vi "SMO.StopDependencies.vi"(8 "error in (no error)":errorcluster, 11 "SMO in":refnum<class "SMO.lvclass">) -> (0 "error out":errorcluster, 3 "SMO out":refnum<class "SMO.lvclass">)   [LabVIEW 2021, in "smo.lvlib" / "SMO.lvclass"]
uses:
  SMO.lvclass
  SMO.lvclass/SMO.ctl
  Typedefs/SMO Dependency Event--Cluster.ctl
  Typedefs/SMO Dependency Event--Enum.ctl
  GetVariant(Attr).vi
  ReftoDVR--SMO.vi
  Support/Attribute.Dependencies/Attribute.Dependencies.lvclass
  C:/Repositories/SMO/src/Support/Attribute/Attribute.lvclass
  Support/Attribute.Dependencies/Get GUIDs.vi
  Support/Attribute.Dependencies/Initialize Dependencies Attribute.vi
  UpdateAttribute.vi
  <vilib>/Utility/MD5Checksum.llb/MD5Checksum string.vi
  Support/Attribute.Owner/Attribute.Owner.lvclass
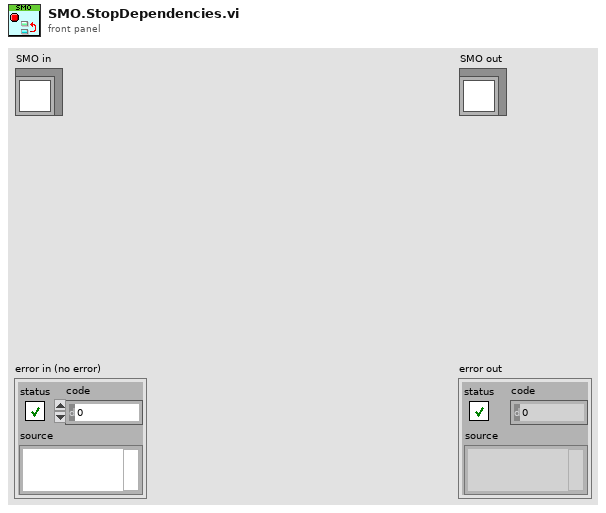
[diagram p1: front panel]
types:
  T1 = typedef "smo.lvlib/Attribute.Dependencies.lvclass/DependencyAttr--Cluster.ctl" = cluster{"Name":string, "GUID":string, "owned":bool, "shared":bool, "Level":string, "SMO":refnum<class "SMO.lvclass">}
  T2 = typedef "smo.lvlib/SMO.lvclass/SMO Dependency Event--Cluster.ctl" = cluster{"Name":string, "GUID":string, "Event":T3}
  T3 = typedef "smo.lvlib/SMO.lvclass/SMO Dependency Event--Enum.ctl" = enum16{"Added", "Removed", "Started", "Stopped"}
  T4 = typedef "smo.lvlib/SMO.lvclass/Protected Events.ctl" = cluster{"StopProcesses":refnum<user-event>, "AbortProcesses":refnum<user-event>, "Config Changed":refnum<user-event>, "Dependency":refnum<user-event>}
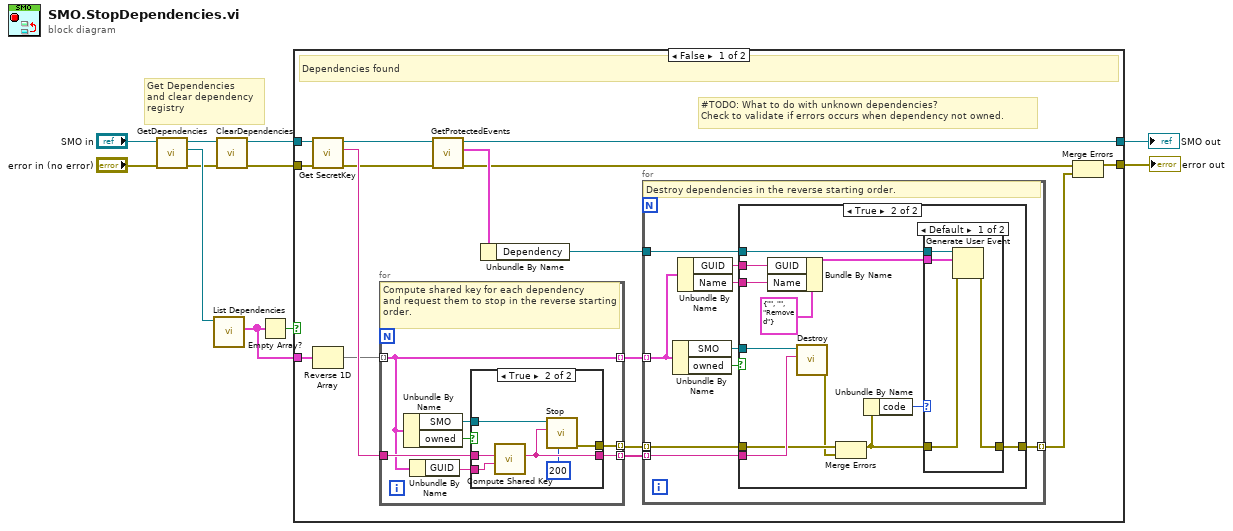
[diagram p0: block diagram]
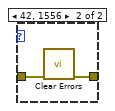
[diagram p3: hidden frame]
diagram:
  # "Get Dependencies\nand clear dependency\nregistry"
  n1 = call "GetDependencies.vi"("error in (no error)"="error in (no error)", "SMO in"="SMO in") -> ("error out"=w6:errorcluster, "Dependencies"=w10:refnum<class "Attribute.Dependencies.lvclass">, "SMO out"=w8:refnum<class "SMO.lvclass">)  [unwired: 7 in]
  n2 = call "List Dependencies.vi"("Attribute.Dependencies in"=w10) -> ("Dependencies"=w9:T1[])  [unwired: 8 in, 2 out]
  n3 = call "ClearDependencies.vi"("error in (no error)"=w6, "SMO in"=w8) -> ("error out"=w5:errorcluster, "SMO out"=w7:refnum<class "SMO.lvclass">)  [unwired: 8 in]
  n4 = Empty Array?(array=w9) -> (empty?=w11:bool)
  n5 = case shown="False" w11 {
    tunnel: [w27 w69] -> w2
    tunnel: w9 -> [w26 _]
    tunnel: w7 -> [w25 w70]
    tunnel: [w19 w70] -> w3
    tunnel: w5 -> [w18 w69]
    frame False {
      # "#TODO: What to do with unknown dependencies?\nCheck to validate if errors occurs when dependency not owned."
      # "Dependencies found"
      n6 = call "Get SecretKey.vi"("error in (no error)"=w18, "SMO"=w25) -> ("error out"=w17:errorcluster, "SecretKey"=w24:string, "SMO out"=w22:refnum<class "SMO.lvclass">)  [unwired: 7 in]
      n7 = Reverse 1D Array(array=w26) -> (reversed array=w15:T1[])
      n8 = for {
        tunnel: w15 -> [w56] mode=indexing
        tunnel: w24 -> [w62]
        tunnel: [w61] -> w23 mode=indexing
        tunnel: [w58] -> w12 mode=indexing
        tunnel: [w56] -> w14 mode=indexing
        # "Compute shared key for each dependency\nand request them to stop in the reverse starting\norder."
        n9 = Unbundle By Name(w56) -> ("SMO"=w59:refnum<class "SMO.lvclass">, "owned"=w60:bool)
        n10 = Unbundle By Name(w56) -> ("GUID"=w57:string)
        n11 = case shown="True" w60 {
          tunnel: w62 -> [_ w68]
          tunnel: [_ w65] -> w61
          tunnel: w57 -> [_ w67]
          tunnel: w59 -> [_ w66]
          tunnel: [_ w64] -> w58
          frame False {
          }
          frame True {
            n12 = call "Compute Shared Key.vi"("GUID"=w67, "SecretKey"=w68) -> ("Shared Key"=w65:string)  [unwired: 9 in]
            n13 = call "Stop.vi"("timeout in ms (-1)"=200, "Shared Key"=w65, "SMO"=w66) -> ("error out"=w64:errorcluster)  [unwired: 7 in, 1 out]
          }
        }
      }
      n14 = call "GetProtectedEvents.vi"("error in (no error)"=w17, "SMO"=w22) -> ("error out"=w16:errorcluster, "SMO Protected Events"=w21:T4, "SMO out"=w19:refnum<class "SMO.lvclass">)  [unwired: 7 in]
      n15 = Unbundle By Name(w21) -> ("Dependency"=w20:refnum<user-event>)
      n16 = for {
        tunnel: w23 -> [w36] mode=indexing
        tunnel: [w35] -> w13 mode=indexing
        tunnel: w20 -> [w32]
        tunnel: w14 -> [w31] mode=indexing
        tunnel: w12 -> [w28] mode=indexing
        # "Destroy dependencies in the reverse starting order."
        n17 = Unbundle By Name(w31) -> ("SMO"=w34:refnum<class "SMO.lvclass">, "owned"=w33:bool)
        n18 = Unbundle By Name(w31) -> ("GUID"=w30:string, "Name"=w29:string)
        n19 = case shown="True" w33 {
          tunnel: w36 -> [_ w49]
          tunnel: [w37 w47] -> w35
          tunnel: w32 -> [_ w44]
          tunnel: w34 -> [_ w46]
          tunnel: w30 -> [_ w42]
          tunnel: w29 -> [_ w41]
          tunnel: w28 -> [w37 w40]
          frame False {
          }
          frame True {
            n20 = Bundle By Name(cluster=T2 {"Name"="", "GUID"="", "Event"=enum."Removed"} ("Dependency Event"), "GUID"=w42, "Name"=w41) -> (w43:T2)
            n21 = call "Destroy.vi"("Shared Key"=w49, "SMO"=w46) -> ("error out"=w39:errorcluster)  [unwired: 9 in]
            n22 = Merge Errors(w40, w39) -> (w38:errorcluster)
            n23 = Unbundle By Name(w38) -> ("code"=w48:i32)
            n24 = case shown="Default" w48 {
              tunnel: w38 -> [w51 w55]
              tunnel: [w50 w54] -> w47
              tunnel: w43 -> [w52 _]
              tunnel: w44 -> [w53 _]
              frame Default {
                n25 = Generate User Event(user event=w53, event data cluster=w52, error in=w51) -> (error out=w50:errorcluster)  [unwired: 1 in, 1 out]
              }
              frame 42, 1556 {
                n26 = call <vilib>:"Clear Errors.vi"("error in (no error)"=w55) -> ("error out"=w54:errorcluster)  [unwired: 5 in, 1 out]
              }
            }
          }
        }
      }
      n27 = Merge Errors(w16, w13) -> (w27:errorcluster)
    }
    frame True {
      # "No dependencies found"
    }
  }
  "error out" <- w2
  "SMO out" <- w3
